vi "SaveScanSettings.vi"(3 "Type of scan":T12=enum."M scan", 4 "Digitizer Settings":T4={"Digitizer delay (us) "=0.0, "rf points per line"=2048, "lines per plane"=128, "Samp Rate (Hz)"=100000000.0, "Additional dig delay (us)"=0.0, "Voltage Scale"=0.4, "Pre-Looks"=0, "Offset delay (us)"=0.0, "bits A/D"=8, "Avg Num"=1, "DigTimeOut"=5.0, "Rel Dig Delay"=0.0, "Dig Ch"=0, "LeCroyCluster"={"LeCroy Channels"=[TRUE, FALSE, FALSE, FALSE], "LC read pt offset"=0.0, "Sweep Avg"=FALSE}, "Main Digitizer"=enum."NI Digitizer", "Dig Config"=enum."Single channel", "Digitizer ID Cluster"={"Acqiris/Alazar/SP ID"=[], "NI Instr Handles"=[], "LeCroy VISA"="", "GaGe Handle"={"Handle"=0, "Sample size"=0, "Resolution"=0, "Offset"=0, "Channels"=0, "Boards"=0}, "ATS Ref"="ATS9350", "Acqiris Address"=["PCI::INSTR0"], "ADQRef"=refnum, "adq_cu_ptr"=refnum}, "Trigger Settings"={"Trig Source"=1, "Trig Coupling"=0, "Trig Slope"=0, "Level (mV)"=1500.0}, "Bulk Acq"=FALSE, "Bulk Start Indexes"=[], "Data Ref RF"=refnum, "NI ID/Channel"=[], "Total Dig CH"=1, "Xtra Ann Trig delay (us)"=10.0, "Fix Z Delay?"=FALSE, "One Way Transmission?"=FALSE, "Data Ref Log"=refnum} {"Trigger Settings"."Trig Slope" items=["Positive", "Negative"]; "Trigger Settings"."Level (mV)" format="%.2f"; "Trigger Settings"."Trig Coupling" items=["DC 1 MOhm", "AC 1 MOhm", "DC 50 Ohm", "AC 50 Ohm"]; "Trigger Settings"."Trig Source" items=["Chan 1", "External"]; "Rel Dig Delay" format="%.2f"; "DigTimeOut" format="%.2f"; "Avg Num" min=1; "Offset delay (us)" format="%.2f"; "Additional dig delay (us)" format="%.2f"; "Digitizer delay (us)" format="%.2f"}, 5 "Motion Settings":T8={"No Motion?"=FALSE, "Motion System"=enum."NI 735x", "Motion Bd ID"=1, "Motion Profile"="SMAC1", "# Axis"=1, "Reverse Z axis?"=TRUE, "SMAC Axis"=0, "scan pair"=enum."x-(y) scan", "RT fps"=6.0, "Steps per mm"=[1000, 1000, 1000, 1000], "Motor Parameters"={"velocity ct/s"=[10000.0, 10000.0, 10000.0, 50000.0], "accel ct/s^2"=[50000.0, 50000.0, 50000.0, 200000.0]}, "One Way Scan"=FALSE, "Reverse One Way Scan"=FALSE, "Global Position (mm)"=[], "Plane"=0, "Distance between\nscan lines (um)"=0.0, "Distance between\nscan planes (um)"=0.0, "number of scan planes"=1, "Total steps in line"=0, "Xtra plane\ndistance  (um)"=100, "Xtra planes "=1, "Add Axis"=FALSE, "overshoot cts"=200, "BKPT Shift"=0, "Scan Start Time (ms)"=0, "ESP VISA"="GPIB::1::INSTR", "3rd Axis"=1, "GL Ref Out"=refnum, "Galil Address"=""} {"3rd Axis" items=["x", "y", "z", "w"]; "Xtra planes" min=1; "Xtra plane\ndistance  (um)" min=0; "Distance between\nscan planes (um)" format="%.2f"; "Distance between\nscan lines (um)" format="%.2f"; "SMAC Axis" items=["None"=0, "Axis 1"=1, "Axis 2"=2, "Axis 3"=3, "Axis 4"=4, "Axis 5"=5, "Axis 6"=6, "Axis 7"=7, "Axis 8"=8, "Vector Space 1"=17, "Vector Space 2"=18, "Vector Space 3"=19, "Vector Space 4"=20]; "Motion Bd ID" min=1 max=32 step=1}, 6 "Case Name Modifier":string="Case") -> (0 "Type of scan out":T12=enum."M scan", 1 "Digitizer Settings out":T4={"Digitizer delay (us) "=0.0, "rf points per line"=2048, "lines per plane"=128, "Samp Rate (Hz)"=100000000.0, "Additional dig delay (us)"=0.0, "Voltage Scale"=0.4, "Pre-Looks"=0, "Offset delay (us)"=0.0, "bits A/D"=8, "Avg Num"=1, "DigTimeOut"=5.0, "Rel Dig Delay"=0.0, "Dig Ch"=0, "LeCroyCluster"={"LeCroy Channels"=[TRUE, FALSE, FALSE, FALSE], "LC read pt offset"=0.0, "Sweep Avg"=FALSE}, "Main Digitizer"=enum."NI Digitizer", "Dig Config"=enum."Single channel", "Digitizer ID Cluster"={"Acqiris/Alazar/SP ID"=[], "NI Instr Handles"=[], "LeCroy VISA"="", "GaGe Handle"={"Handle"=0, "Sample size"=0, "Resolution"=0, "Offset"=0, "Channels"=0, "Boards"=0}, "ATS Ref"="ATS9350", "Acqiris Address"=["PCI::INSTR0"], "ADQRef"=refnum, "adq_cu_ptr"=refnum}, "Trigger Settings"={"Trig Source"=1, "Trig Coupling"=0, "Trig Slope"=0, "Level (mV)"=1500.0}, "Bulk Acq"=FALSE, "Bulk Start Indexes"=[], "Data Ref RF"=refnum, "NI ID/Channel"=[], "Total Dig CH"=5, "Xtra Ann Trig delay (us)"=10.0, "Fix Z Delay?"=FALSE, "One Way Transmission?"=FALSE, "Data Ref Log"=refnum} {"Trigger Settings"."Trig Slope" items=["Positive", "Negative"]; "Trigger Settings"."Level (mV)" format="%.2f"; "Trigger Settings"."Trig Coupling" items=["DC 1 MOhm", "AC 1 MOhm", "DC 50 Ohm", "AC 50 Ohm"]; "Trigger Settings"."Trig Source" items=["Chan 1", "External"]; "Rel Dig Delay" format="%.2f"; "DigTimeOut" format="%.2f"; "Avg Num" min=1; "Offset delay (us)" format="%.2f"; "Additional dig delay (us)" format="%.2f"; "Digitizer delay (us)" format="%.2f"}, 2 "Motion Settings out":T8={"No Motion?"=FALSE, "Motion System"=enum."NI 735x", "Motion Bd ID"=1, "Motion Profile"="SMAC1", "# Axis"=1, "Reverse Z axis?"=TRUE, "SMAC Axis"=0, "scan pair"=enum."y-(x) scan", "RT fps"=6.0, "Steps per mm"=[1000, 1000, 1000, 1000], "Motor Parameters"={"velocity ct/s"=[10000.0, 10000.0, 10000.0, 50000.0], "accel ct/s^2"=[50000.0, 50000.0, 50000.0, 200000.0]}, "One Way Scan"=FALSE, "Reverse One Way Scan"=FALSE, "Global Position (mm)"=[], "Plane"=0, "Distance between\nscan lines (um)"=0.0, "Distance between\nscan planes (um)"=0.0, "number of scan planes"=1, "Total steps in line"=0, "Xtra plane\ndistance  (um)"=100, "Xtra planes "=1, "Add Axis"=FALSE, "overshoot cts"=200, "BKPT Shift"=0, "Scan Start Time (ms)"=0, "ESP VISA"="GPIB::1::INSTR", "3rd Axis"=1, "GL Ref Out"=refnum, "Galil Address"=""} {"3rd Axis" items=["x", "y", "z", "w"]; "Xtra planes" min=1; "Xtra plane\ndistance  (um)" min=0; "Distance between\nscan planes (um)" format="%.2f"; "Distance between\nscan lines (um)" format="%.2f"; "SMAC Axis" items=["None"=0, "Axis 1"=1, "Axis 2"=2, "Axis 3"=3, "Axis 4"=4, "Axis 5"=5, "Axis 6"=6, "Axis 7"=7, "Axis 8"=8, "Vector Space 1"=17, "Vector Space 2"=18, "Vector Space 3"=19, "Vector Space 4"=20]; "Motion Bd ID" min=1 max=32 step=1})   [LabVIEW 2022 SP3]
uses:
  Controls/CompleteScanSettings.ctl
  Controls/ScanType2.ctl
  Motion Controllers/NI_controller/-NI_MotionRoutines/MotionParameters.ctl
  Motion Controllers/NI_controller/-NI_MotionRoutines/MotionSys.ctl
  Motion Controllers/-MotionRoutines/ScanAxis.ctl
  Motion Controllers/-MotionRoutines/3rdAxis.ctl
  Digitizers/-DigitizerRoutines/DigitizerSettings.ctl
  Digitizers/-DigitizerRoutines/Digitizer.ctl
  Digitizers/-DigitizerRoutines/DigConfig.ctl
  Digitizers/-DigitizerRoutines/DigitizerID.ctl
  C:/Windows/System32/ADQAPI_dotNet_helper.dll
  Pulsers/Panametrics/Pana5900.ctl
  Pulsers/Daxsonics/-DaxSubroutines/Dax_Control_Cluster.ctl
  Pulsers/pulser.ctl
  Motion Controllers/-MotionRoutines/MotionGlobals.vi
  <vilib>/Utility/xml.llb/Write to XML File(string).vi
  Pulsers/PulserGlobals.vi
panel:
  in  "Cancel":bool
  out "error out":errorcluster
  in  "Daxsonics Settings":T1={"Freq (MHz) "=20, "Voltage (V)"=0, "Gain (dB)"=22} {"Freq (MHz)" items=["50"=50, "45"=45, "40"=40, "35"=35, "30"=30, "25"=25, "20"=20, "18"=18, "17"=17, "16"=16, "15"=15, "14"=14, "12"=12, "10"=10, "8"=8, "6"=6, "5"=5, "4"=4]; "Voltage (V)" items=["190"=190, "180"=180, "170"=170, "160"=160, "150"=150, "140"=140, "130"=130, "120"=120, "110"=110, "100"=100, "95"=95, "90"=90, "85"=85, "80"=80, "75"=75, "70"=70, "65"=65, "60"=60, "55"=55, "50"=50, "45"=45, "40"=40, "35"=35, "30"=30, "25"=25, "20"=20, "15"=15, "10"=10, "5"=5, "0"=0]; "Gain (dB)" items=["67"=67, "64"=64, "61"=61, "58"=58, "55"=55, "52"=52, "49"=49, "46"=46, "43"=43, "40"=40, "37"=37, "34"=34, "31"=31, "28"=28, "25"=25, "22"=22]}
  in  "Panametrics Settings":T2={"ENERGY (uJ)"=0, "DAMPING (Ohm)"=0, "HP FILT (KHz) "=0, "LP FILT (MHz)"=0, "MODE"=0, "PRF (KHz)"=1, "GAIN (db)"=0, "COARSE ATTENUATION"=0, "FINE ATTENUATION"=0} {"FINE ATTENUATION" items=["00.0", "00.5", "01.0", "01.5", "02.0", "02.5", "03.0", "03.5", "04.0", "04.5", "05.0", "05.5", "06.0", "06.5", "07.0", "07.5", "08.0", "08.5", "09.0", "09.5", "10.0", "10.5", "11.0", "11.5", "12.0", "12.5", "13.0", "13.5", "14.0", "14.5", "15.0", "15.5"]; "COARSE ATTENUATION" items=["00.0", "10.0", "20.0", "30.0", "40.0", "50.0"]; "GAIN (db)" items=["26.0", "40.0", "54.0"]; "PRF (KHz)" items=["XREMT", "EXBNC", "0.200", "0.500", "1.000", "2.000", "5.000", "10.00", "20.00"]; "MODE" items=["P/ E", "THRU", "RPP", "EXT_PLSR"]; "LP FILT (MHz)" items=["20", "50", "100", "200"]; "HP FILT (KHz)" items=["1", "1000", "3000", "10000"]; "DAMPING (Ohm)" items=["7", "10", "16", "20", "26", "30", "40", "50"]; "ENERGY (uJ)" items=["1", "2", "4", "8", "16", "32"]}
  in  "Pulser":T3
  out "Size of one \nRF line (mm)":dbl=128.0 format="%.2f"
  out "Size of all \nplanes (mm)":dbl=128.0 format="%.2f"
  out "Size of one \nplane (mm)":dbl=128.0 format="%.2f"
  in  "Fix Z Delay?":bool
  in  "Voltage Scale":dbl
  in  "Additional dig delay (us)":dbl
  in  "Digitizer delay (us)":dbl
  in  "Samp Rate (MHz)":dbl
  in  "lines per plane":i32
  in  "rf points per line":i32
  in  "number of scan planes":i32
  in  "Distance between\nscan planes (um)":sgl
  in  "Distance between\nscan lines (um)":sgl
  in  "Reverse One Way Scan":bool
  in  "One Way Scan":bool
  in  "scan pair":T10=enum."x-(y) scan"
  in  "save":bool
  in  "ScanSettings":T13={"Type of scan"=enum."M scan", "Motion Settings In"={"No Motion?"=FALSE, "Motion System"=enum."NI 735x", "Motion Bd ID"=1, "Motion Profile"="SMAC1", "# Axis"=1, "Reverse Z axis?"=TRUE, "SMAC Axis"=0, "scan pair"=enum."y-(x) scan", "RT fps"=6.0, "Steps per mm"=[1000, 1000, 1000, 1000], "Motor Parameters"={"velocity ct/s"=[10000.0, 10000.0, 10000.0, 50000.0], "accel ct/s^2"=[50000.0, 50000.0, 50000.0, 200000.0]}, "One Way Scan"=FALSE, "Reverse One Way Scan"=FALSE, "Global Position (mm)"=[], "Plane"=0, "Distance between\nscan lines (um)"=0.0, "Distance between\nscan planes (um)"=0.0, "number of scan planes"=1, "Total steps in line"=0, "Xtra plane\ndistance  (um)"=100, "Xtra planes "=1, "Add Axis"=FALSE, "overshoot cts"=200, "BKPT Shift"=0, "Scan Start Time (ms)"=0, "ESP VISA"="GPIB::1::INSTR", "3rd Axis"=1, "GL Ref Out"=refnum, "Galil Address"=""}, "Digitizer Settings"={"Digitizer delay (us) "=0.0, "rf points per line"=2048, "lines per plane"=128, "Samp Rate (Hz)"=100000000.0, "Additional dig delay (us)"=0.0, "Voltage Scale"=0.4, "Pre-Looks"=0, "Offset delay (us)"=0.0, "bits A/D"=8, "Avg Num"=1, "DigTimeOut"=5.0, "Rel Dig Delay"=0.0, "Dig Ch"=0, "LeCroyCluster"={"LeCroy Channels"=[TRUE, FALSE, FALSE, FALSE], "LC read pt offset"=0.0, "Sweep Avg"=FALSE}, "Main Digitizer"=enum."NI Digitizer", "Dig Config"=enum."Single channel", "Digitizer ID Cluster"={"Acqiris/Alazar/SP ID"=[], "NI Instr Handles"=[], "LeCroy VISA"="", "GaGe Handle"={"Handle"=0, "Sample size"=0, "Resolution"=0, "Offset"=0, "Channels"=0, "Boards"=0}, "ATS Ref"="ATS9350", "Acqiris Address"=["PCI::INSTR0"], "ADQRef"=refnum, "adq_cu_ptr"=refnum}, "Trigger Settings"={"Trig Source"=1, "Trig Coupling"=0, "Trig Slope"=0, "Level (mV)"=1500.0}, "Bulk Acq"=FALSE, "Bulk Start Indexes"=[], "Data Ref RF"=refnum, "NI ID/Channel"=[], "Total Dig CH"=1, "Xtra Ann Trig delay (us)"=10.0, "Fix Z Delay?"=FALSE, "One Way Transmission?"=FALSE, "Data Ref Log"=refnum}, "Case Name Modifier"="Case", "Panametrics Settings"={"ENERGY (uJ)"=0, "DAMPING (Ohm)"=0, "HP FILT (KHz) "=0, "LP FILT (MHz)"=0, "MODE"=0, "PRF (KHz)"=1, "GAIN (db)"=0, "COARSE ATTENUATION"=0, "FINE ATTENUATION"=0}, "Daxsonics Settings"={"Freq (MHz) "=20, "Voltage (V)"=0, "Gain (dB)"=22}, "Pulser"=enum."Pan 5900"} {"Daxsonics Settings"."Freq (MHz)" items=["50"=50, "45"=45, "40"=40, "35"=35, "30"=30, "25"=25, "20"=20, "18"=18, "17"=17, "16"=16, "15"=15, "14"=14, "12"=12, "10"=10, "8"=8, "6"=6, "5"=5, "4"=4]; "Daxsonics Settings"."Voltage (V)" items=["190"=190, "180"=180, "170"=170, "160"=160, "150"=150, "140"=140, "130"=130, "120"=120, "110"=110, "100"=100, "95"=95, "90"=90, "85"=85, "80"=80, "75"=75, "70"=70, "65"=65, "60"=60, "55"=55, "50"=50, "45"=45, "40"=40, "35"=35, "30"=30, "25"=25, "20"=20, "15"=15, "10"=10, "5"=5, "0"=0]; "Daxsonics Settings"."Gain (dB)" items=["67"=67, "64"=64, "61"=61, "58"=58, "55"=55, "52"=52, "49"=49, "46"=46, "43"=43, "40"=40, "37"=37, "34"=34, "31"=31, "28"=28, "25"=25, "22"=22]; "Panametrics Settings"."FINE ATTENUATION" items=["00.0", "00.5", "01.0", "01.5", "02.0", "02.5", "03.0", "03.5", "04.0", "04.5", "05.0", "05.5", "06.0", "06.5", "07.0", "07.5", "08.0", "08.5", "09.0", "09.5", "10.0", "10.5", "11.0", "11.5", "12.0", "12.5", "13.0", "13.5", "14.0", "14.5", "15.0", "15.5"]; "Panametrics Settings"."COARSE ATTENUATION" items=["00.0", "10.0", "20.0", "30.0", "40.0", "50.0"]; "Panametrics Settings"."GAIN (db)" items=["26.0", "40.0", "54.0"]; "Panametrics Settings"."PRF (KHz)" items=["XREMT", "EXBNC", "0.200", "0.500", "1.000", "2.000", "5.000", "10.00", "20.00"]; "Panametrics Settings"."MODE" items=["P/ E", "THRU", "RPP", "EXT_PLSR"]; "Panametrics Settings"."LP FILT (MHz)" items=["20", "50", "100", "200"]; "Panametrics Settings"."HP FILT (KHz)" items=["1", "1000", "3000", "10000"]; "Panametrics Settings"."DAMPING (Ohm)" items=["7", "10", "16", "20", "26", "30", "40", "50"]; "Panametrics Settings"."ENERGY (uJ)" items=["1", "2", "4", "8", "16", "32"]; "Digitizer Settings"."Trigger Settings"."Trig Slope" items=["Positive", "Negative"]; "Digitizer Settings"."Trigger Settings"."Level (mV)" format="%.2f"; "Digitizer Settings"."Trigger Settings"."Trig Coupling" items=["DC 1 MOhm", "AC 1 MOhm", "DC 50 Ohm", "AC 50 Ohm"]; "Digitizer Settings"."Trigger Settings"."Trig Source" items=["Chan 1", "External"]; "Digitizer Settings"."Rel Dig Delay" format="%.2f"; "Digitizer Settings"."DigTimeOut" format="%.2f"; "Digitizer Settings"."Avg Num" min=1; "Digitizer Settings"."Offset delay (us)" format="%.2f"; "Digitizer Settings"."Additional dig delay (us)" format="%.2f"; "Digitizer Settings"."Digitizer delay (us)" format="%.2f"; "Motion Settings In"."3rd Axis" items=["x", "y", "z", "w"]; "Motion Settings In"."Xtra planes" min=1; "Motion Settings In"."Xtra plane\ndistance  (um)" min=0; "Motion Settings In"."Distance between\nscan planes (um)" format="%.2f"; "Motion Settings In"."Distance between\nscan lines (um)" format="%.2f"; "Motion Settings In"."SMAC Axis" items=["None"=0, "Axis 1"=1, "Axis 2"=2, "Axis 3"=3, "Axis 4"=4, "Axis 5"=5, "Axis 6"=6, "Axis 7"=7, "Axis 8"=8, "Vector Space 1"=17, "Vector Space 2"=18, "Vector Space 3"=19, "Vector Space 4"=20]; "Motion Settings In"."Motion Bd ID" min=1 max=32 step=1}
  # "Confirm Relevant Settings"
  # "1-D and 2-D B scan settings"
  # "1-D and 2-D B scan settings"
  # "1-D and 2-D B scan settings"
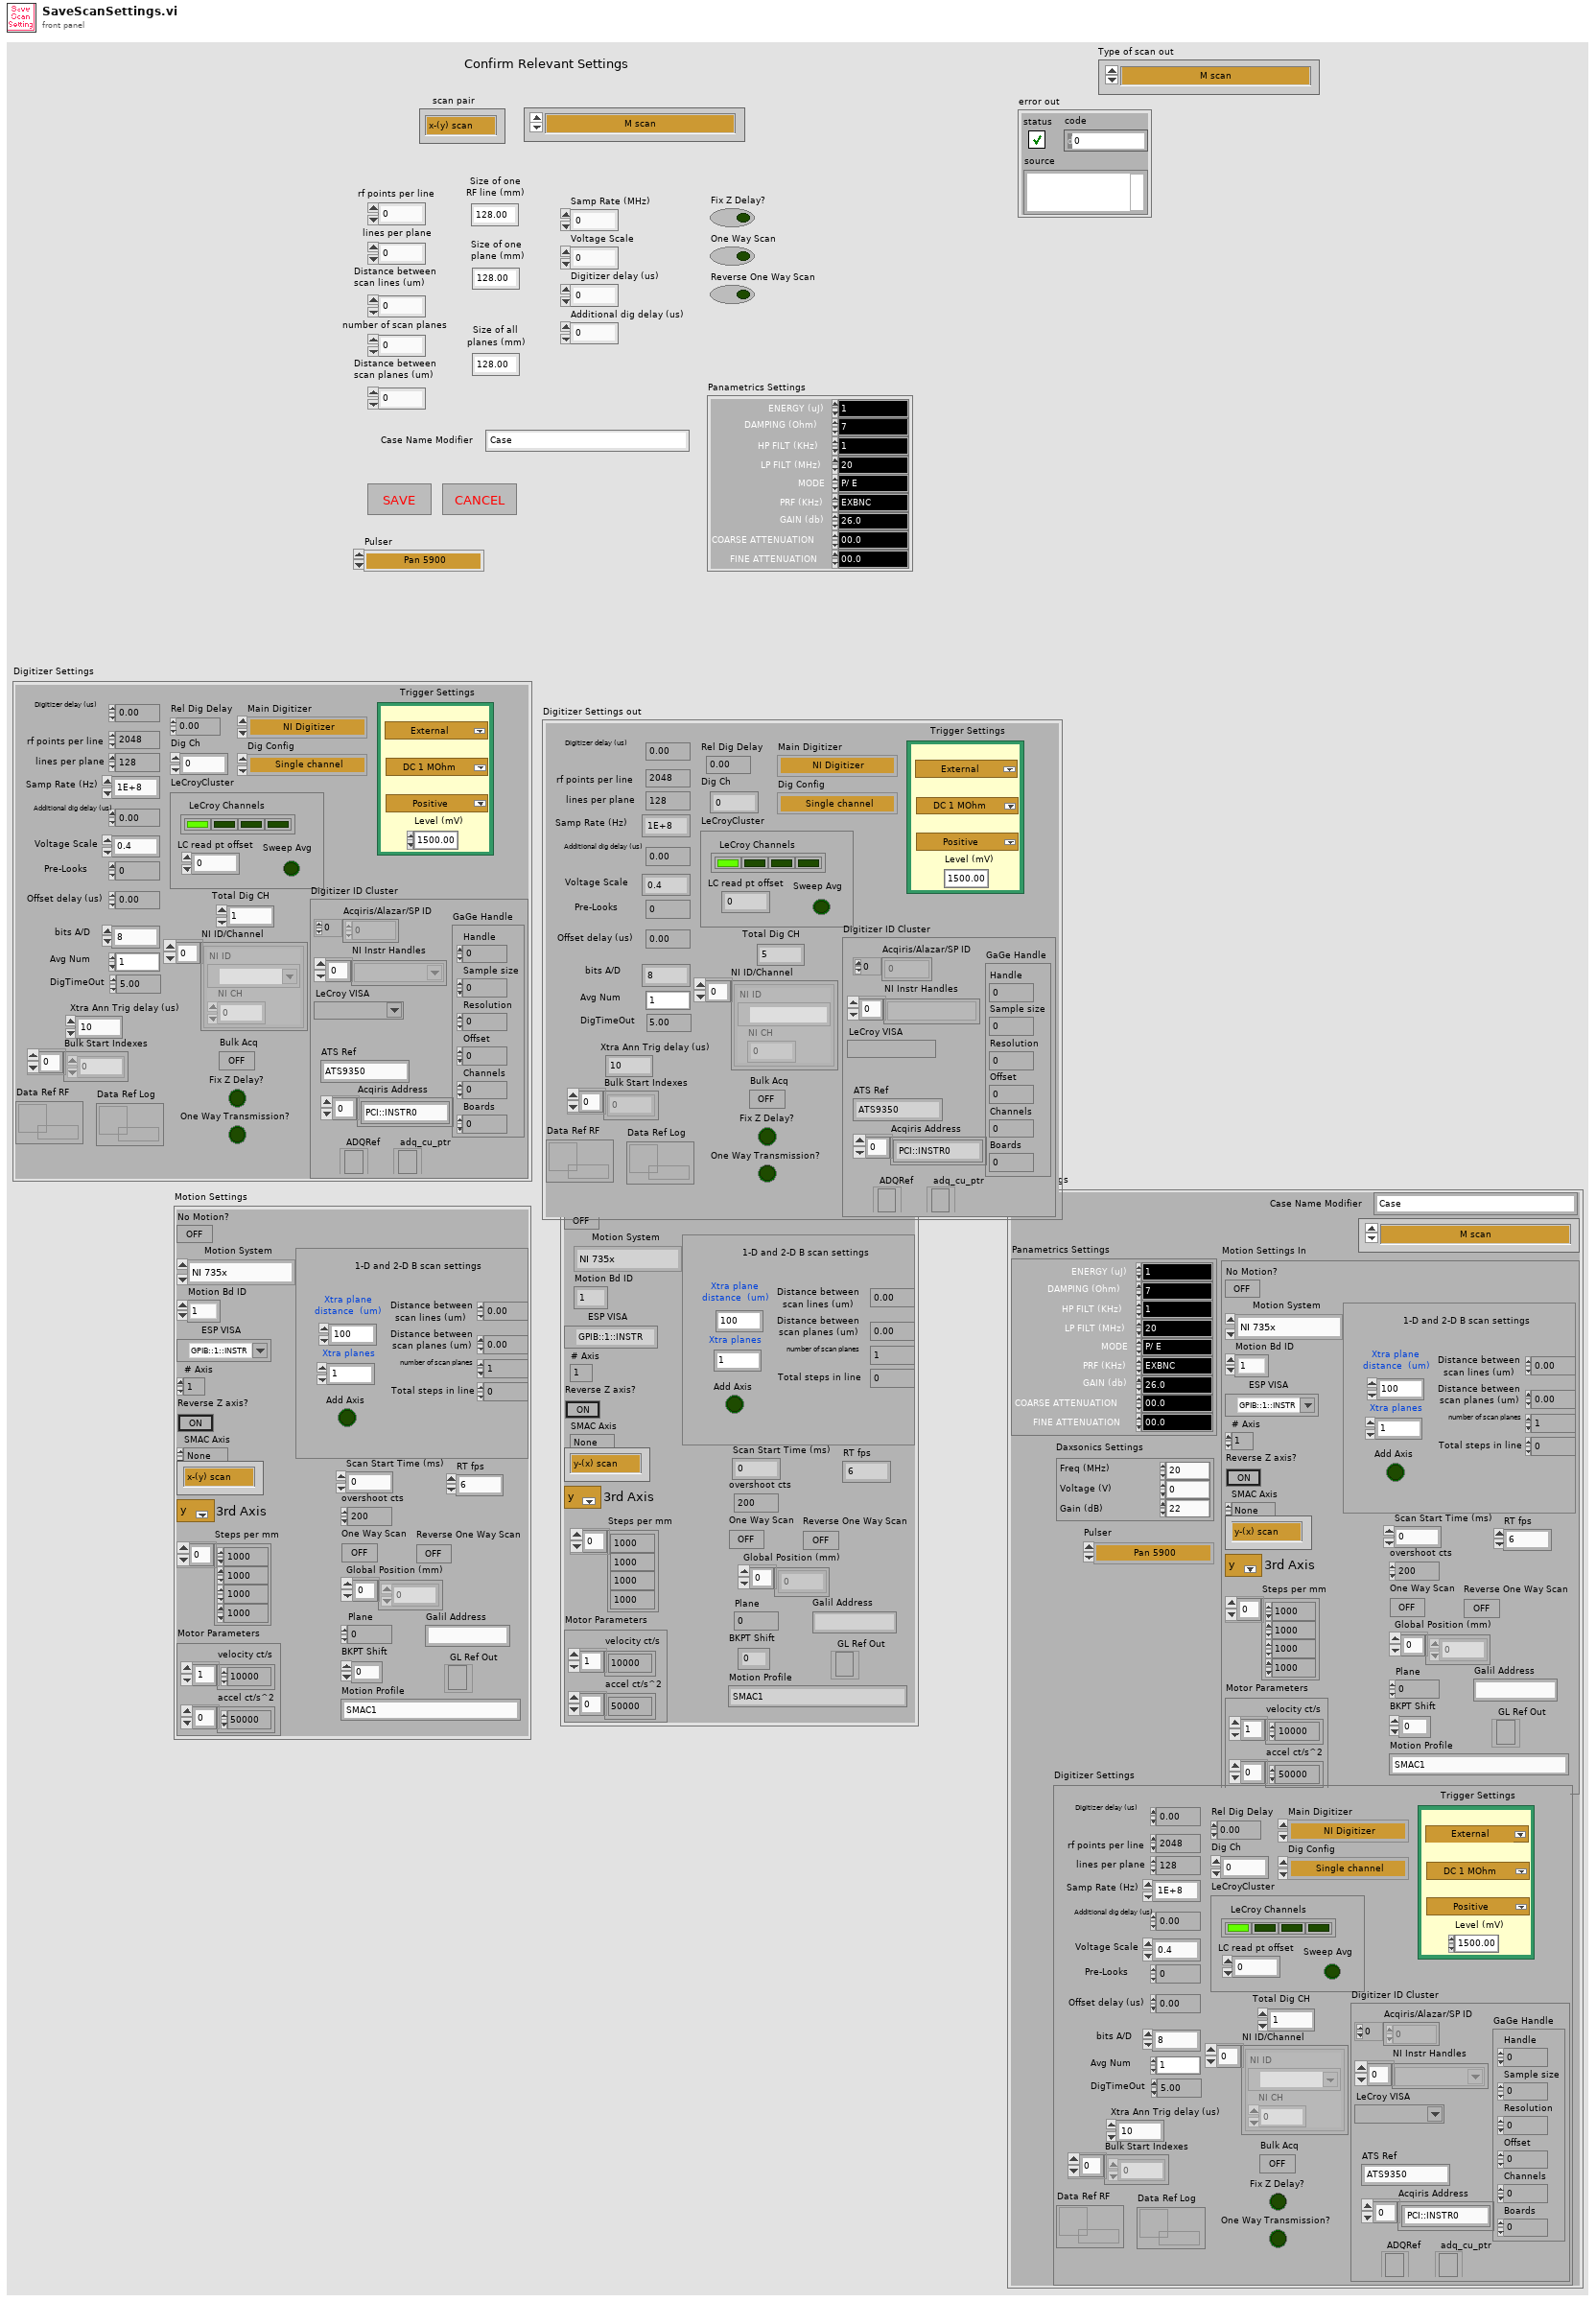
[diagram p1: front panel]
types:
  T1 = typedef "Dax_Control_Cluster.ctl" = cluster{"Freq (MHz) ":u16, "Voltage (V)":u16, "Gain (dB)":u16}
  T2 = typedef "Pana5900.ctl" = cluster{"ENERGY (uJ)":u16, "DAMPING (Ohm)":u16, "HP FILT (KHz) ":u16, "LP FILT (MHz)":u16, "MODE":u16, "PRF (KHz)":u16, "GAIN (db)":u16, "COARSE ATTENUATION":u16, "FINE ATTENUATION":u16}
  T3 = typedef "pulser.ctl" = enum16{"Pan 5900", "Daxsonics", "Agilent 33xxx", "UTEX", "JSR", "WMC Mono-Cycle", "No Pulser", "NYU AVTECH", "Tabor W1281A", "Pan 5800", "Unlisted", "Tabor WX2182B"}
  T4 = typedef "DigitizerSettings.ctl" = cluster{"Digitizer delay (us) ":dbl, "rf points per line":i32, "lines per plane":i32, "Samp Rate (Hz)":dbl, "Additional dig delay (us)":dbl, "Voltage Scale":dbl, "Pre-Looks":i32, "Offset delay (us)":dbl, "bits A/D":i8, "Avg Num":i32, "DigTimeOut":sgl, "Rel Dig Delay":sgl, "Dig Ch":i32, "LeCroyCluster":cluster{"LeCroy Channels":bool[], "LC read pt offset":dbl, "Sweep Avg":bool}, "Main Digitizer":T5, "Dig Config":T6, "Digitizer ID Cluster":T7, "Trigger Settings":cluster{"Trig Source":u16, "Trig Coupling":u16, "Trig Slope":u16, "Level (mV)":dbl}, "Bulk Acq":bool, "Bulk Start Indexes":i32[], "Data Ref RF":refnum<data-value>, "NI ID/Channel":cluster{"NI ID":refnum<k15>, "NI CH":i32}[], "Total Dig CH":i32, "Xtra Ann Trig delay (us)":dbl, "Fix Z Delay?":bool, "One Way Transmission?":bool, "Data Ref Log":refnum<data-value>}
  T5 = typedef "Digitizer.ctl" = enum16{"Acqiris Digitizer", "NI Digitizer", "LeCroy", "GaGe", "AlazarTech", "No Digitizer", "Teledyne"}
  T6 = typedef "DigConfig.ctl" = enum16{"Single channel", "2 Chans w/ 2 Acqiris", "2 Chans w/ 1 Acqiris", "5-CH Pulser New", "5-CH pulser w/ ann array", "5-pass style ann array", "Empty"}
  T7 = typedef "DigitizerID.ctl" = cluster{"Acqiris/Alazar/SP ID":u32[], "NI Instr Handles":refnum<k15>[], "LeCroy VISA":refnum<visa-resource-name>, "GaGe Handle":cluster{"Handle":u32, "Sample size":u32, "Resolution":i32, "Offset":i32, "Channels":u32, "Boards":u32}, "ATS Ref":string, "Acqiris Address":string[], "ADQRef":refnum<k24>, "adq_cu_ptr":refnum<k24>}
  T8 = typedef "MotionParameters.ctl" = cluster{"No Motion?":bool, "Motion System":T9, "Motion Bd ID":u8, "Motion Profile":string, "# Axis":i8, "Reverse Z axis?":bool, "SMAC Axis":u16, "scan pair":T10, "RT fps":sgl, "Steps per mm":i32[], "Motor Parameters":cluster{"velocity ct/s":dbl[], "accel ct/s^2":dbl[]}, "One Way Scan":bool, "Reverse One Way Scan":bool, "Global Position (mm)":dbl[], "Plane":i32, "Distance between\nscan lines (um)":sgl, "Distance between\nscan planes (um)":sgl, "number of scan planes":i32, "Total steps in line":i32, "Xtra plane\ndistance  (um)":i32, "Xtra planes ":i32, "Add Axis":bool, "overshoot cts":i32, "BKPT Shift":i32, "Scan Start Time (ms)":u32, "ESP VISA":refnum<visa-resource-name>, "3rd Axis":T11, "GL Ref Out":refnum<k7>, "Galil Address":string}
  T9 = typedef "MotionSys.ctl" = enum16{"MM3000", "NI 735x", "Newport ESP", "No Motion Card", "Galil"}
  T10 = typedef "ScanAxis.ctl" = enum16{"y-(x) scan", "x-(y) scan", "z-(x) scan", "z-(y) scan", "y-(z) scan", "x-(z) scan", "w-(x) scan", "w-(y) scan", "w-(z) scan", "x-(w) scan", "y-(w) scan", "z-(w) scan"}
  T11 = typedef "3rdAxis.ctl" = u16
  T12 = typedef "ScanType2.ctl" = enum16{"Therapy With Scan", "M scan", "M Scan With Therapy Burst", "1-D B Scan", "1-D B Scan With Therapy Burst", "2-D B Scan", "2-D B Scan With Therapy Burst", "Rotational Scan", "1-D B-Scan PRF", "2-D B-Scan PRF", "Real-Time Scan", "Contrast Agents", "1-D w/ Real-Time Set Up", "Dual Transducer", "Acoustic Microscopy", "Hydrophone Scanning"}
  T13 = typedef "CompleteScanSettings.ctl" = cluster{"Type of scan":T12, "Motion Settings In":T8, "Digitizer Settings":T4, "Case Name Modifier":string, "Panametrics Settings":T2, "Daxsonics Settings":T1, "Pulser":T3}
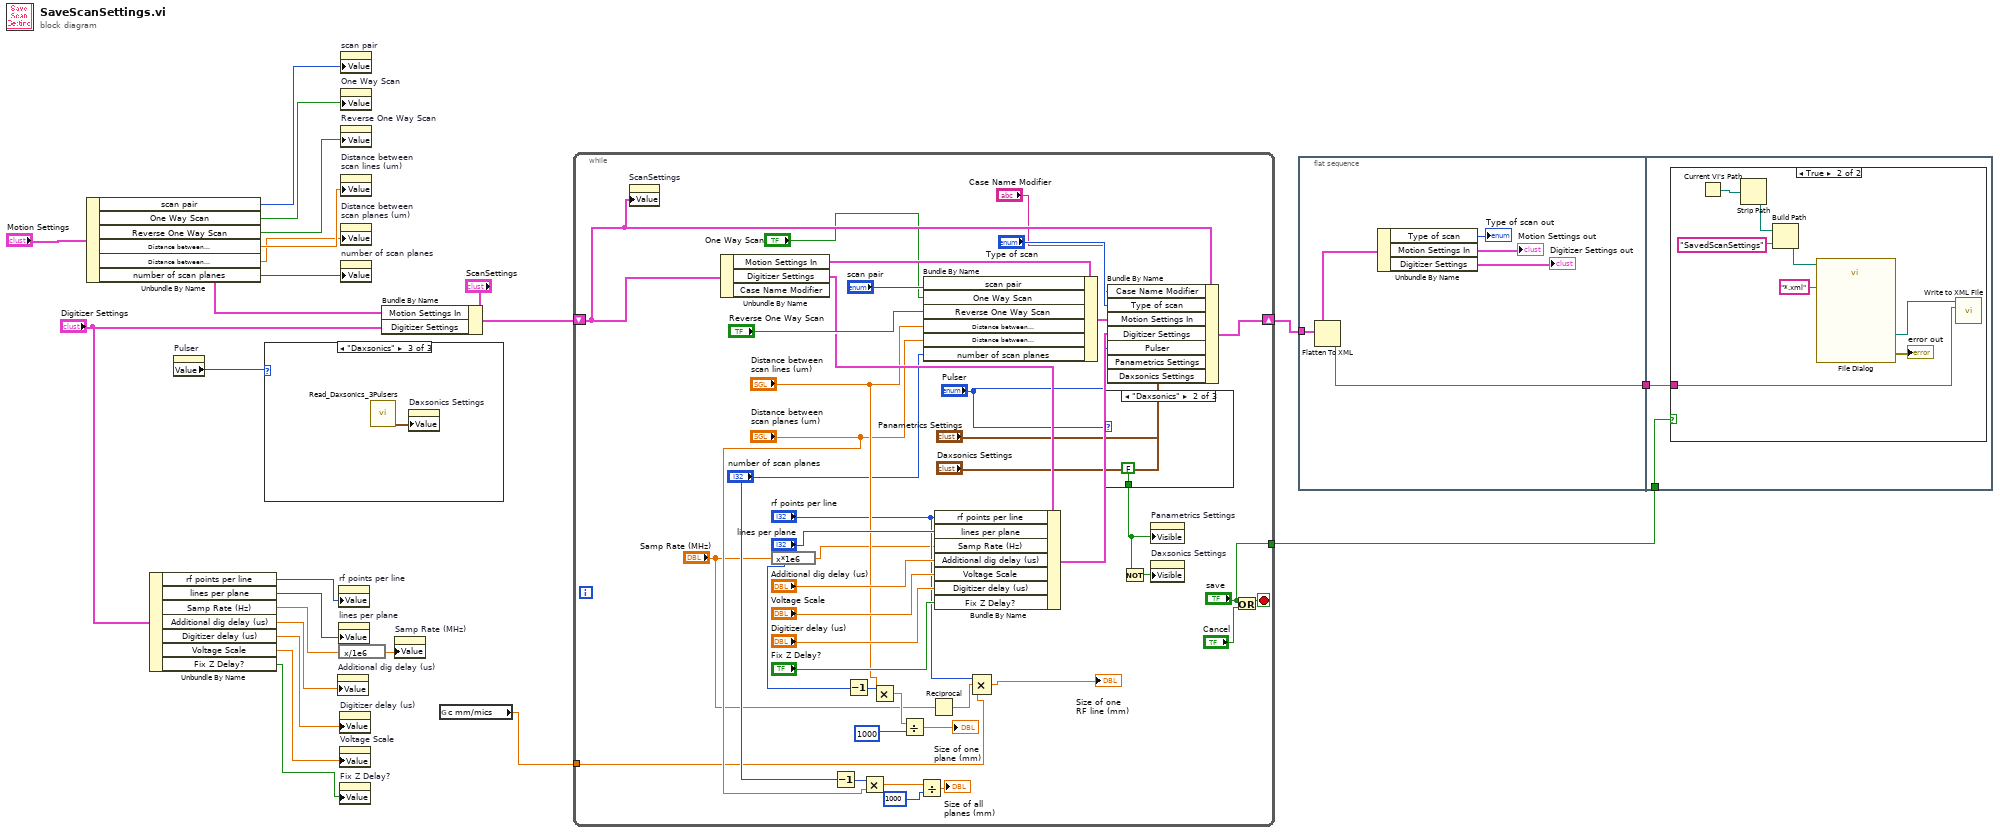
[diagram p0: block diagram]
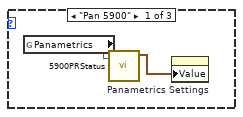
[diagram p3: hidden frame]
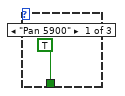
[diagram p5: hidden frame]
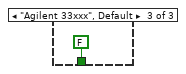
[diagram p6: hidden frame]
diagram:
  n1 = Unbundle By Name("Motion Settings") -> ("scan pair"=w21:T10, "One Way Scan"=w20:bool, "Reverse One Way Scan"=w19:bool, "Distance between\nscan lines (um)"=w18:sgl, "Distance between\nscan planes (um)"=w17:sgl, "number of scan planes"=w16:i32)
  n2 = Unbundle By Name("Digitizer Settings") -> ("rf points per line"=w15:i32, "lines per plane"=w14:i32, "Samp Rate (Hz)"=w13:dbl, "Additional dig delay (us)"=w11:dbl, "Digitizer delay (us)"=w10:dbl, "Voltage Scale"=w9:dbl, "Fix Z Delay?"=w8:bool)
  n3 = property on="Pulser" class="Enum (strict)"() -> ("Value"=w3:T3)  [unwired: 2 in, 2 out]
  n4 = case shown="\"Daxsonics\"" w3 {
    frame "Pan 5900" {
      n5 = global read "PulserGlobals.vi" "Panametrics"() -> (w24:refnum<visa-resource-name>)
      n6 = call "5900PRStatus.vi"("VISA resource name"=w24) -> ("Panametrics Settings"=w25:T2)  [unwired: 1 in, 3 out]
      n7 = property on="Panametrics Settings" class="Clust (strict)"("Value"=w25) -> ()  [unwired: 2 in, 2 out]
    }
    frame "Agilent 33xxx", Default {
    }
    frame "Daxsonics" {
      n8 = call "Read_Daxsonics_3Pulsers.vi"() -> ("Dax Values"=w26:T1)  [unwired: 5 in, 6 out]
      n9 = property on="Daxsonics Settings" class="Clust (strict)"("Value"=w26) -> ()  [unwired: 2 in, 2 out]
    }
  }
  n10 = property on="Additional dig delay (us)" class="DigNum (strict)"("Value"=w11) -> ()  [unwired: 2 in, 2 out]
  n11 = property on="rf points per line" class="DigNum (strict)"("Value"=w15) -> ()  [unwired: 2 in, 2 out]
  n12 = property on="lines per plane" class="DigNum (strict)"("Value"=w14) -> ()  [unwired: 2 in, 2 out]
  n13 = expression code="x/1e6"(w13) -> (w12:dbl)
  n14 = property on="Digitizer delay (us)" class="DigNum (strict)"("Value"=w10) -> ()  [unwired: 2 in, 2 out]
  n15 = property on="Voltage Scale" class="DigNum (strict)"("Value"=w9) -> ()  [unwired: 2 in, 2 out]
  n16 = property on="Fix Z Delay?" class="Bool (strict)"("Value"=w8) -> ()  [unwired: 2 in, 2 out]
  n17 = property on="scan pair" class="Enum (strict)"("Value"=w21) -> ()  [unwired: 2 in, 2 out]
  n18 = property on="One Way Scan" class="Bool (strict)"("Value"=w20) -> ()  [unwired: 2 in, 2 out]
  n19 = property on="Reverse One Way Scan" class="Bool (strict)"("Value"=w19) -> ()  [unwired: 2 in, 2 out]
  n20 = property on="Distance between\nscan lines (um)" class="DigNum (strict)"("Value"=w18) -> ()  [unwired: 2 in, 2 out]
  n21 = property on="Distance between\nscan planes (um)" class="DigNum (strict)"("Value"=w17) -> ()  [unwired: 2 in, 2 out]
  n22 = property on="number of scan planes" class="DigNum (strict)"("Value"=w16) -> ()  [unwired: 2 in, 2 out]
  n23 = Bundle By Name(cluster="ScanSettings", "Motion Settings In"="Motion Settings", "Digitizer Settings"="Digitizer Settings") -> (w22:T13)
  n24 = property on="Samp Rate (MHz)" class="DigNum (strict)"("Value"=w12) -> ()  [unwired: 2 in, 2 out]
  n25 = global read "MotionGlobals.vi" "c mm/mics"() -> (w4:sgl)
  n26 = while {
    shift-right: [w66] -> w5
    shift-left: w22 -> [w67]
    tunnel: w4 -> [w37]
    tunnel: ["save"] -> w1
    stop <- w30 stop-if-true
    n27 = property on="ScanSettings" class="Clust (strict)"("Value"=w67) -> ()  [unwired: 2 in, 2 out]
    n28 = Unbundle By Name(w67) -> ("Motion Settings In"=w65:T8, "Digitizer Settings"=w60:T4)  [unwired: 1 out]
    n29 = expression code="x*1e6"("Samp Rate (MHz)") -> (w39:dbl)
    n30 = Decrement(x="number of scan planes") -> (x-1=w47:i32)
    n31 = Decrement(x="lines per plane") -> (x-1=w52:i32)
    n32 = Multiply(x=w47, y="Distance between\nscan planes (um)") -> (x*y=w46:sgl)
    n33 = Multiply(x=w52, y="Distance between\nscan lines (um)") -> (x*y=w49:sgl)
    n34 = Divide(x=w49, y=1000 ("x")) -> (x/y=→"Size of one \nplane (mm)":sgl)
    n35 = Divide(x=w46, y=1000 ("x")) -> (x/y=→"Size of all \nplanes (mm)":sgl)
    n36 = Bundle By Name(cluster=w65, "scan pair"="scan pair", "One Way Scan"="One Way Scan", "Reverse One Way Scan"="Reverse One Way Scan", "Distance between\nscan lines (um)"="Distance between\nscan lines (um)", "Distance between\nscan planes (um)"="Distance between\nscan planes (um)", "number of scan planes"="number of scan planes") -> (w64:T8)
    n37 = Reciprocal(x="Samp Rate (MHz)") -> (1/x=w40:dbl)
    n38 = Bundle By Name(cluster=w60, "rf points per line"="rf points per line", "lines per plane"="lines per plane", "Samp Rate (Hz)"=w39, "Additional dig delay (us)"="Additional dig delay (us)", "Voltage Scale"="Voltage Scale", "Digitizer delay (us)"="Digitizer delay (us)", "Fix Z Delay?"="Fix Z Delay?") -> (w59:T4)
    n39 = Compound Arithmetic op=MULTIPLY("rf points per line", w40, w37) -> (→"Size of one \nRF line (mm)":dbl)
    n40 = case shown="\"Daxsonics\"" "Pulser" {
      tunnel: [TRUE FALSE FALSE] -> w35
      frame "Pan 5900" {
      }
      frame "Daxsonics" {
      }
      frame "Agilent 33xxx", Default {
      }
    }
    n41 = Bundle By Name(cluster=w67, "Case Name Modifier"="Case Name Modifier", "Type of scan"="Type of scan", "Motion Settings In"=w64, "Digitizer Settings"=w59, "Pulser"="Pulser", "Panametrics Settings"="Panametrics Settings", "Daxsonics Settings"="Daxsonics Settings") -> (w66:T13)
    n42 = Not(x=w35) -> (.not. x?=w34:bool)
    n43 = property on="Panametrics Settings" class="Clust (strict)"("Visible"=w35) -> ()  [unwired: 2 in, 2 out]
    n44 = property on="Daxsonics Settings" class="Clust (strict)"("Visible"=w34) -> ()  [unwired: 2 in, 2 out]
    n45 = Or(x="save", y="Cancel") -> (x .or. y?=w30:bool)
  }
  n46 = flat-sequence {
    tunnel: w5 -> [w74]
    tunnel: [w75] -> w2
    tunnel: w2 -> [w77]
    tunnel: w1 -> [w76]
    frame #0 {
      n47 = Flatten To XML(6:w74) -> (2:w75:string)
      n48 = Unbundle By Name(w74) -> ("Type of scan"=→"Type of scan out":T12, "Motion Settings In"=→"Motion Settings out":T8, "Digitizer Settings"=→"Digitizer Settings out":T4)
    }
    frame #1 {
      n49 = case shown="True" w76 {
        tunnel: w77 -> [_ w81]
        frame False {
        }
        frame True {
          n50 = Current VI's Path() -> (path=w83:path)
          n51 = Strip Path(path=w83) -> (stripped path=w79:path)  [unwired: 1 out]
          n52 = Build Path(base path=w79, name or relative path="SavedScanSettings") -> (appended path=w84:path)
          n53 = call "File Dialog"("start path"=w84, "pattern (all files)"="*.xml") -> ("selected path"=w82:path, "error out"=→"error out":errorcluster)  [unwired: 10 in, 2 out]
          n54 = call-poly <vilib>:"Write to XML File.vi"("XML Input"=w81, "XML File Path"=w82) -> ()  [unwired: 7 in, 3 out]
        }
      }
    }
  }
